vi "SetParameter.vi"(8 "error in (no error)":errorcluster, 10 "SetParameter":T1, 11 "NHRDCPower in":refnum<class "NHRDCPower.lvclass">) -> (0 "error out":errorcluster, 2 "StatusUpdates":string[](array[string]), 3 "NHRDCPower out":refnum<class "NHRDCPower.lvclass">)   [LabVIEW 2018, in "AcPwrPlugins.lvlib" / "NHRDCPower.lvclass"]
uses:
  NHRDCPower.lvclass
  AcPwrBaseClass/TypeDefs/SetParameterInputs.ctl
  AcPwrBaseClass/AcPwrBase.lvclass
  <instrlib>/NHRDCPowerModule/NHRDCPowerModule/NHRDCPowerModule.lvlib
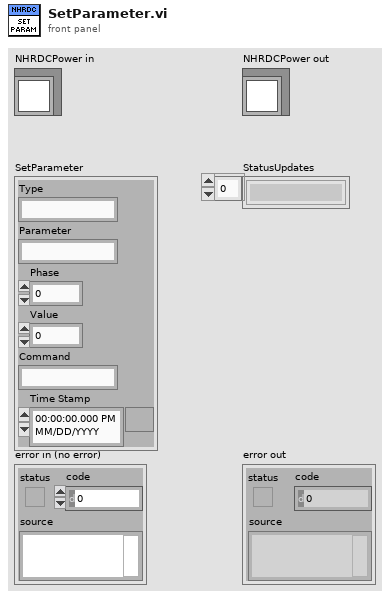
[diagram p1: front panel]
types:
  T1 = typedef "AcPwrPlugins.lvlib/AcPwrBase.lvclass/SetParameterInputs.ctl" = cluster{"Type":string, "Parameter":string, "Phase":i32, "Value":dbl, "Command":string, "Time Stamp":timestamp}
  T2 = typedef "AcPwrPlugins.lvlib/NHRDCPower.lvclass/Modules.ctl" = cluster{"Handle":string, "Name":string, "id query (Yes)":bool, "reset device (Yes)":bool, "Connected":bool, "Initial Battery Detect Voltage (0)":dbl, "SafetySettings":cluster{"SetWatchDog?":bool, "Voltage (V)":dbl, "Current (A)":dbl, "Power (W)":dbl, "Voltage Delay (s)":dbl, "Current Delay (s)":dbl, "Power Delay (s)":dbl}, "Options String":string, "Aperture Time (s)":dbl, "operating state (Off)":i32, "OutputSettings":cluster{"Voltage (V)":dbl, "Current (A)":dbl, "Resistance (Ohms)":dbl, "Power (W)":dbl, "Enable Voltage":bool, "Enable Current":bool, "Enable Resistance":bool, "Enable Power":bool, "Macro After Step Delay  (s)":dbl, "Wait Value (V, A, W)":dbl, "Enable Wait":bool, "Wait on Value":i32}[], "SlewRate":cluster{"Set Voltage Rate V/S":dbl, "Set Current Rate A/S":dbl, "Set Resistance Rate R/S":dbl, "Set Power Rate W/S":dbl}, "Macro":cluster{"Save Macro?":bool, "Load Macro From File?":bool, "Run Macro Continuously?":bool, "Use Macros?":bool, "Load Macro File Path":string, "Save Macro File Path":string}, "Regulation Gain (1=100%)":dbl, "UpdatingOntheFly":bool}[]
  T3 = cluster{"Handle":string, "Name":string, "id query (Yes)":bool, "reset device (Yes)":bool, "Connected":bool, "Initial Battery Detect Voltage (0)":dbl, "SafetySettings":cluster{"SetWatchDog?":bool, "Voltage (V)":dbl, "Current (A)":dbl, "Power (W)":dbl, "Voltage Delay (s)":dbl, "Current Delay (s)":dbl, "Power Delay (s)":dbl}, "Options String":string, "Aperture Time (s)":dbl, "operating state (Off)":i32, "OutputSettings":cluster{"Voltage (V)":dbl, "Current (A)":dbl, "Resistance (Ohms)":dbl, "Power (W)":dbl, "Enable Voltage":bool, "Enable Current":bool, "Enable Resistance":bool, "Enable Power":bool, "Macro After Step Delay  (s)":dbl, "Wait Value (V, A, W)":dbl, "Enable Wait":bool, "Wait on Value":i32}[], "SlewRate":cluster{"Set Voltage Rate V/S":dbl, "Set Current Rate A/S":dbl, "Set Resistance Rate R/S":dbl, "Set Power Rate W/S":dbl}, "Macro":cluster{"Save Macro?":bool, "Load Macro From File?":bool, "Run Macro Continuously?":bool, "Use Macros?":bool, "Load Macro File Path":string, "Save Macro File Path":string}, "Regulation Gain (1=100%)":dbl, "UpdatingOntheFly":bool}
  T4 = cluster{"Handle":string, "Name":string, "id query (Yes)":bool, "reset device (Yes)":bool, "Connected":bool, "Initial Battery Detect Voltage (0)":dbl, "SafetySettings":cluster{"SetWatchDog?":bool, "Voltage (V)":dbl, "Current (A)":dbl, "Power (W)":dbl, "Voltage Delay (s)":dbl, "Current Delay (s)":dbl, "Power Delay (s)":dbl}, "Options String":string, "Aperture Time (s)":dbl, "operating state (Off)":i32, "OutputSettings":cluster{"Voltage (V)":dbl, "Current (A)":dbl, "Resistance (Ohms)":dbl, "Power (W)":dbl, "Enable Voltage":bool, "Enable Current":bool, "Enable Resistance":bool, "Enable Power":bool, "Macro After Step Delay  (s)":dbl, "Wait Value (V, A, W)":dbl, "Enable Wait":bool, "Wait on Value":i32}[], "SlewRate":cluster{"Set Voltage Rate V/S":dbl, "Set Current Rate A/S":dbl, "Set Resistance Rate R/S":dbl, "Set Power Rate W/S":dbl}, "Macro":cluster{"Save Macro?":bool, "Load Macro From File?":bool, "Run Macro Continuously?":bool, "Use Macros?":bool, "Load Macro File Path":string, "Save Macro File Path":string}, "Regulation Gain (1=100%)":dbl, "UpdatingOntheFly":bool}[]
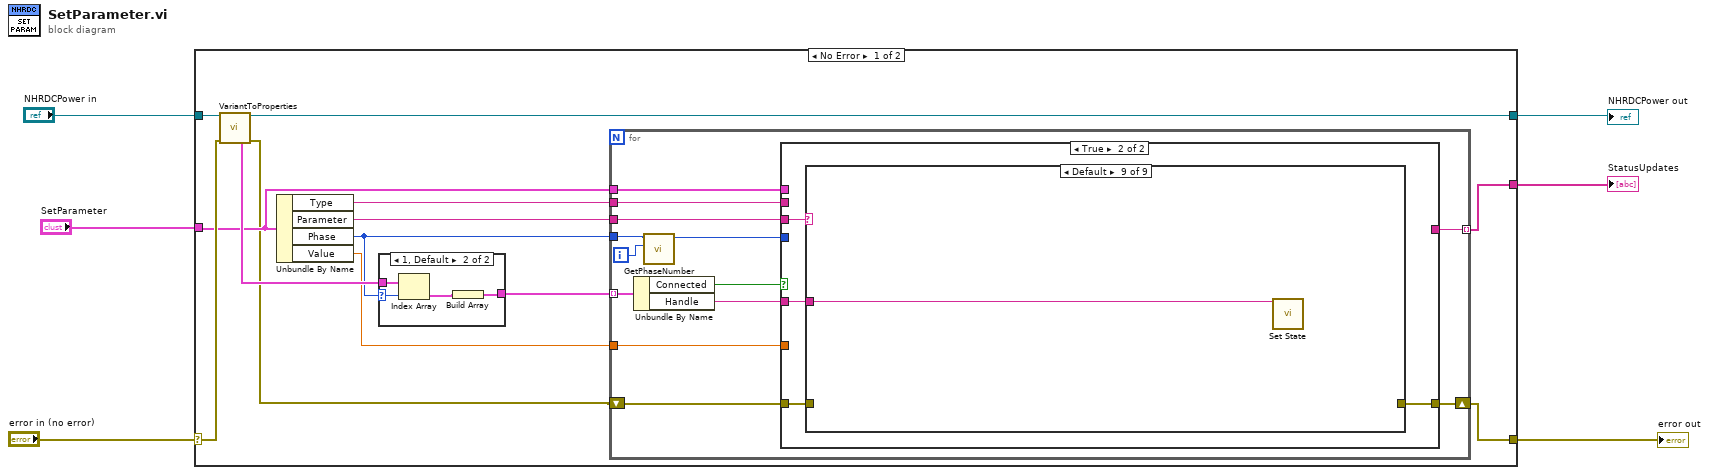
[diagram p0: block diagram]
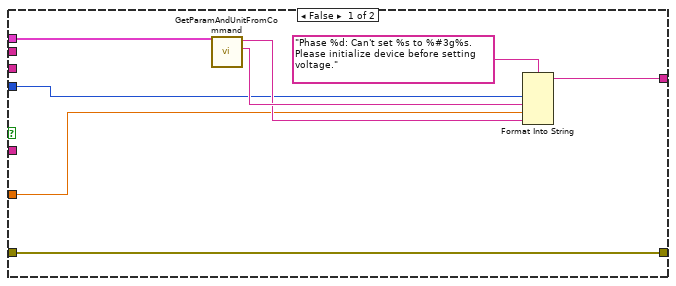
[diagram p2: hidden frame]
diagram:
  n1 = case shown="No Error" "error in (no error)" {
    selector: "error in (no error)" -> [w18 w52]
    tunnel: "NHRDCPower in" -> [w19 w53]
    tunnel: [w16 w53] -> w4
    tunnel: [w7 w52] -> w3
    tunnel: [w8 _] -> w2
    tunnel: "SetParameter" -> [w12 _]
    frame No Error {
      n2 = call "VariantToProperties.vi"("NHRDCPower in"=w19, "error in (no error)"=w18) -> ("NHRDCPower out"=w16:refnum<class "NHRDCPower.lvclass">, "Modules"=w17:T2, "error out"=w10:errorcluster)  [unwired: 7 in, 4 out]
      n3 = Unbundle By Name(w12) -> ("Type"=w15:string, "Parameter"=w14:string, "Phase"=w13:i32, "Value"=w9:dbl)
      n4 = case shown="1, Default" w13 {
        selector: w13 -> [_ w51]
        tunnel: w17 -> [w47 w50]
        tunnel: [w47 w48] -> w11
        frame -1 {
        }
        frame 1, Default {
          n5 = Index Array(array=w50, index=w51) -> (element=w49:T3)
          n6 = Build Array(w49) -> (w48:T4)
        }
      }
      n7 = for {
        tunnel: w15 -> [w27]
        tunnel: w14 -> [w26]
        tunnel: w13 -> [w32]
        tunnel: w12 -> [w28]
        tunnel: w11 -> [w30] mode=indexing
        shift-right: [w20] -> w7
        shift-left: w10 -> [w23]
        tunnel: w9 -> [w22]
        tunnel: [w21] -> w8 mode=indexing
        i -> [w31]
        n8 = Unbundle By Name(w30) -> ("Connected"=w29:bool, "Handle"=w24:string)
        n9 = call "GetPhaseNumber.vi"("Loop Counter"=w31, "Phase(-1, all) in"=w32) -> ("Phase(-1, all) out"=w25:i32)  [unwired: 9 in]
        n10 = case shown="True" w29 {
          tunnel: w28 -> [w37 _]
          tunnel: w27 -> [_ _]
          tunnel: w26 -> [_ w44]
          tunnel: w25 -> [w36 _]
          tunnel: w24 -> [_ w41]
          tunnel: w23 -> [w33 w43]
          tunnel: w22 -> [w35 _]
          tunnel: [w34 _] -> w21
          tunnel: [w33 w42] -> w20
          frame False {
            n11 = call "GetParamAndUnitFromCommand.vi"("SetParameter"=w37) -> ("Parameter"=w39:string, "Unit Label"=w38:string)  [unwired: 9 in]
            n12 = Format Into String(format string="Phase %d: Can't set %s to %#3g%s. Please initialize device before setting voltage.", w36, w39, w35, w38) -> (resulting string=w34:string)  [unwired: 2 in, 1 out]
          }
          frame True {
            n13 = case shown="Default" w44 {
              tunnel: [_ _ _ w45 _ _ _ _ _] -> w42
              tunnel: w43 -> [_ _ _ w45 _ _ _ _ _]
              tunnel: w41 -> [_ _ _ _ _ _ _ _ w46]
              frame "Enable Voltage" {
              }
              frame "Voltage" {
              }
              frame "Enable Current" {
              }
              frame "Current" {
              }
              frame "Enable Resistance" {
              }
              frame "Resistance" {
              }
              frame "Enable Power" {
              }
              frame "Power" {
              }
              frame Default {
                n14 = call <instrlib>:"Set State.vi"("instrument handle"=w46) -> ()  [unwired: 13 in, 2 out]
              }
            }
          }
        }
      }
    }
    frame Error {
    }
  }
  "error out" <- w3
  "NHRDCPower out" <- w4
  "StatusUpdates" <- w2
